vi "PAS Core.vi"(10 "nPAS In":refnum<class "nPAS.lvclass">, 11 "DVR In":refnum<data-value>) -> (3 "nPAS out":refnum<class "nPAS.lvclass">)   [LabVIEW 2016]
uses:
  Data/Nicholas Data.lvclass
  PAS/nPAS.lvclass
  C:/Program Files (x86)/National Instruments/LabVIEW 2016/vi.lib/MSR Consulting, LLC/General Reuse/Instrument/Instrument.lvclass
  <vilib>/MSR Consulting, LLC/General Reuse/Instrument/state.ctl
  <vilib>/MSR Consulting, LLC/General Reuse/Session APIs/Session Log/System Log.lvclass
  C:/Program Files (x86)/National Instruments/LabVIEW 2016/vi.lib/MSR Consulting, LLC/General Reuse/Session APIs/_Session Fwk/Session - Root.lvclass
  <vilib>/MSR Consulting, LLC/General Reuse/Session APIs/File Access/Config Data/Config Data.lvclass
  <vilib>/MSR Consulting, LLC/General Reuse/Session APIs/Session Log/System Log.lvclass/System Log.ctl
  <vilib>/MSR Consulting, LLC/General Reuse/Session APIs/File Access/Config Data/Config Data.lvclass/Config Data.ctl
  <vilib>/MSR Consulting, LLC/General Reuse/Instrument/Instrument.lvclass/Instrument.ctl
  PAS/nPAS.lvclass/nPAS.ctl
  <vilib>/MSR Consulting, LLC/General Reuse/Session APIs/Session Log/Accessors/Write Main Path.vi
  <vilib>/MSR Consulting, LLC/General Reuse/Session APIs/File Access/Config Data/Accessors/Write Cfg Path.vi
  <vilib>/MSR Consulting, LLC/General Reuse/Instrument/Write Log Session.vi
  <vilib>/MSR Consulting, LLC/General Reuse/Instrument/Write Cfg Session.vi
  <vilib>/MSR Consulting, LLC/General Reuse/Instrument/Instrument.lvclass
  <vilib>/MSR Consulting, LLC/General Reuse/Session APIs/_Session Fwk/Session - Root.lvclass
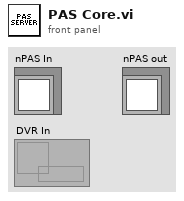
[diagram p1: front panel]
types:
  T1 = typedef "Instrument.lvclass/state.ctl" = enum8{"Configure", "Acquire", "Wait", "Quit", "Handle Error", "NOOP"}
  T2 = typedef "Session - Root.lvclass/Session Handle.ctl" = refnum<data-value>
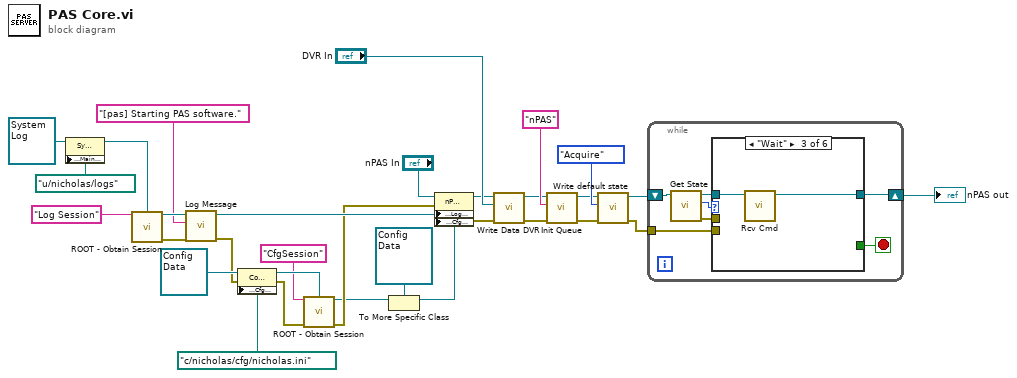
[diagram p0: block diagram]
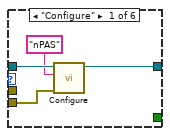
[diagram p2: hidden frame]
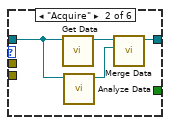
[diagram p3: hidden frame]
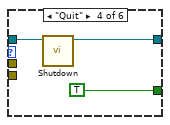
[diagram p4: hidden frame]
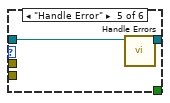
[diagram p5: hidden frame]
diagram:
  n1 = property class="Sys Log"(reference=refnum<class "System Log.lvclass"> refnum ("Sys Log"), "Accessors:Main Path"=path "u:/nicholas/logs" ("Main Path")) -> (reference out=w19:refnum<class "System Log.lvclass">)  [unwired: 1 in, 1 out]
  n2 = call <vilib>:"ROOT - Obtain Session.vi"("Session Name ()"="Log Session", "OBJ - Session"=w19) -> ("Session Handle"=w17:T2, "error out"=w12:errorcluster)  [unwired: 11 in, 1 out]
  n3 = call <vilib>:"Log Message.vi"("error in"=w12, "MSG In"="[pas] Starting PAS software.", "session in"=w17) -> ("error out"=w6:errorcluster, "session out"=w13:T2)  [unwired: 7 in]
  n4 = property class="Config Data"(reference=refnum<class "Config Data.lvclass"> refnum ("Config Data"), error in=w6, "Accessors:Cfg Path"=path "c:/nicholas/cfg/nicholas.ini" ("Cfg Path")) -> (reference out=w9:refnum<class "Config Data.lvclass">, error out=w5:errorcluster)
  n5 = call <vilib>:"ROOT - Obtain Session.vi"("Session Name ()"="CfgSession", "OBJ - Session"=w9, "error in (no error)"=w5) -> ("Session Handle"=w3:T2, "error out"=w7:errorcluster)  [unwired: 10 in, 1 out]
  n6 = To More Specific Class(target class=refnum<data-value> refnum, reference=w3) -> (specific class reference=w2:refnum<data-value>)  [unwired: 1 in, 1 out]
  n7 = property class="nPAS"(reference="nPAS In", error in=w7, "Accessors:Log Session"=w13, "Accessors:Cfg Session"=w2) -> (reference out=w14:refnum<class "nPAS.lvclass">, error out=w4:errorcluster)
  n8 = call "Write Data DVR.vi"("error in (no error)"=w4, "Data DVR"="DVR In", "nPAS in"=w14) -> ("error out"=w22:errorcluster, "nPAS out"=w25:refnum<class "nPAS.lvclass">)  [unwired: 7 in]
  n9 = call <vilib>:"Init Queue.vi"("error in"=w22, "queue_name"="nPAS", "Instrument in"=w25) -> ("error out"=w27:errorcluster, "Instrument out"=w28:refnum<class "nPAS.lvclass">)  [unwired: 7 in]
  n10 = call <vilib>:"Write default state.vi"("error in (no error)"=w27, "instr state"=state."Acquire", "Instrument in"=w28) -> ("error out"=w31:errorcluster, "Instrument out"=w30:refnum<class "nPAS.lvclass">)  [unwired: 7 in]
  n11 = while {
    shift-right: [w36] -> w23
    shift-left: w30 -> [w37]
    tunnel: w31 -> [w35]
    stop <- w38 stop-if-true
    n12 = call <vilib>:"Get State.vi"("Instrument in"=w37) -> ("error out"=w32:errorcluster, "default state"=w34:T1, "Instrument out"=w33:refnum<class "nPAS.lvclass">)  [unwired: 8 in]
    n13 = case shown="\"Wait\"" w34 {
      tunnel: [_ _ _ TRUE _ _] -> w38
      tunnel: w33 -> [w42 w46 w48 w50 w53 w54]
      tunnel: [w41 w45 w47 w49 w52 w54] -> w36
      tunnel: w35 -> [w40 _ _ _ _ _]
      tunnel: w32 -> [_ _ _ _ _ _]
      frame "Configure" {
        n14 = call-dynamic "Configure.vi"("error in"=w40, "name"="nPAS", "nPAS in"=w42) -> ("nPAS out"=w41:refnum<class "nPAS.lvclass">)  [unwired: 7 in, 1 out]
      }
      frame "Acquire" {
        n15 = call-dynamic "Get Data.vi"("nPAS in"=w46) -> ("nPAS out"=w44:refnum<class "nPAS.lvclass">)  [unwired: 9 in, 1 out]
        n16 = call-dynamic "Analyze Data.vi"("nPAS in"=w46) -> ("nPAS out"=w43:refnum<class "nPAS.lvclass">)  [unwired: 9 in, 1 out]
        n17 = call-dynamic "Merge Data.vi"("Analyzed"=w43, "Acquired"=w44) -> ("PAS out"=w45:refnum<class "nPAS.lvclass">)  [unwired: 8 in, 1 out]
      }
      frame "Wait" {
        n18 = call-dynamic "Rcv Cmd.vi"("PAS in"=w48) -> ("PAS out"=w47:refnum<class "nPAS.lvclass">)  [unwired: 9 in, 1 out]
      }
      frame "Quit" {
        n19 = call-dynamic "Shutdown.vi"("nPAS in"=w50) -> ("nPAS out"=w49:refnum<class "nPAS.lvclass">)  [unwired: 9 in, 1 out]
      }
      frame "Handle Error" {
        n20 = call-dynamic "Handle Errors.vi"("Instrument in"=w53) -> ("Instrument out"=w52:refnum<class "nPAS.lvclass">)  [unwired: 8 in, 2 out]
      }
      frame "NOOP", Default {
      }
    }
  }
  "nPAS out" <- w23
